vi "is engine running.vi"(8 "error in":errorcluster, 11 "Standard Engine Runtime in":refnum<class "Standard Engine Runtime.lvclass">) -> (0 "error out":errorcluster, 2 "running?":bool, 3 "Standard Engine Runtime out":refnum<class "Standard Engine Runtime.lvclass">)   [LabVIEW 2013, in "Standard Engine Runtime.lvclass"]
uses:
  Standard Engine Runtime.lvclass
  <vilib>/NI/Module Execution Interface/Engine Runtime/Execution States.ctl
  Standard Engine Runtime.lvclass/Standard Engine Runtime.ctl
  <vilib>/NI/Module Execution Interface/Engine Runtime/Engine Runtime Interface.lvclass
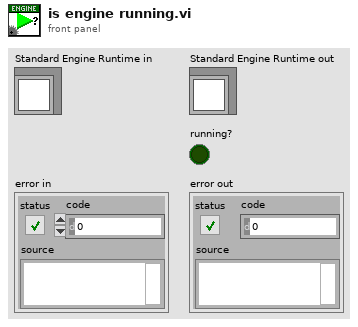
[diagram p1: front panel]
types:
  T1 = typedef "Engine Runtime Interface.lvclass/Execution States.ctl" = enum16{"Init", "Pre-Operational", "Safe-Operational", "Operational", "Stopped"}
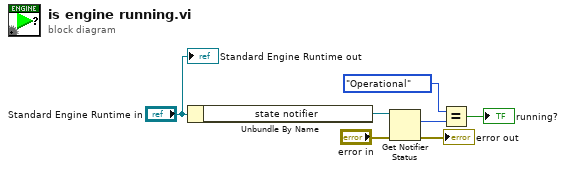
[diagram p0: block diagram]
diagram:
  n1 = Unbundle By Name("Standard Engine Runtime in") -> ("state notifier"=w5:refnum<notifier>)
  n2 = Get Notifier Status(notifier=w5, error in (no error)="error in") -> (current notification=w3:T1, error out=→"error out":errorcluster)  [unwired: 3 out]
  n3 = Equal?(x=Execution_States."Operational" ("latest notification"), y=w3) -> (x = y?=→"running?":bool)
  "Standard Engine Runtime out" <- "Standard Engine Runtime in"
